vi "Stop Live Mode.vi"(7 "Close Viewer":bool=TRUE, 8 "error in (no error)":errorcluster, 10 "Mode":T1, 11 "Application in":refnum<class "Application.lvclass">) -> (0 "error out":errorcluster, 3 "Application out":refnum<class "Application.lvclass">)   [LabVIEW 2023, in "Application.lvlib" / "Application.lvclass"]
uses:
  Application.lvclass
  Application.lvclass/Application.ctl
  Hardware/Camera Messages/Stop Live Mode Msg/Stop Live Mode Msg.lvclass
  Hardware/Sync Device Messages/Stop Streaming Msg/Stop Streaming Msg.lvclass
  Mode.ctl
  Application.lvlib
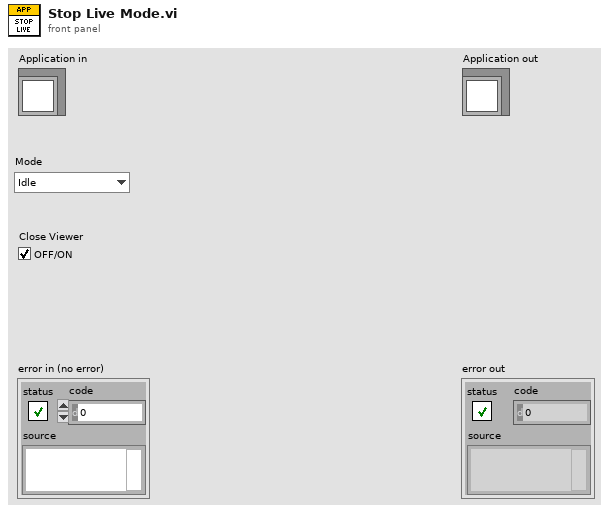
[diagram p1: front panel]
types:
  T1 = typedef "Application.lvlib/Mode.ctl" = enum16{"Idle", "Cancel", "Live", "Stream", "Autofocus", "Z-Stack"}
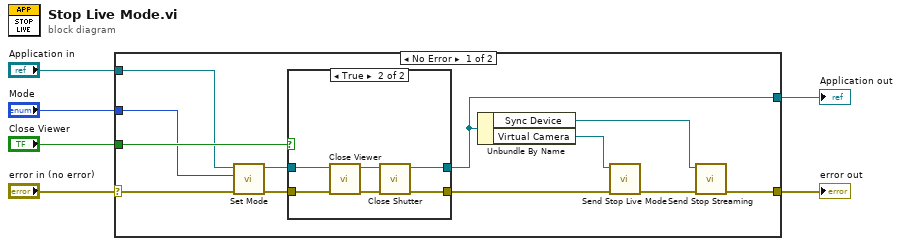
[diagram p0: block diagram]
diagram:
  n1 = case shown="No Error" "error in (no error)" {
    selector: "error in (no error)" -> [w13 w28]
    tunnel: [w9 w28] -> w5
    tunnel: [w17 w27] -> w3
    tunnel: "Application in" -> [w14 w27]
    tunnel: "Close Viewer" -> [w18 _]
    tunnel: "Mode" -> [w12 _]
    frame No Error {
      n2 = call-dynamic "Set Mode.vi"("error in (no error)"=w13, "New Mode"=w12, "Application in"=w14) -> ("error out"=w16:errorcluster, "Application out"=w15:refnum<class "Application.lvclass">)  [unwired: 7 in]
      n3 = case shown="True" w18 {
        tunnel: w16 -> [w19 w26]
        tunnel: w15 -> [w20 w25]
        tunnel: [w20 w22] -> w17
        tunnel: [w19 w21] -> w11
        frame False {
        }
        frame True {
          n4 = call-dynamic "Close Viewer.vi"("error in (no error)"=w26, "Application in"=w25) -> ("error out"=w23:errorcluster, "Application out"=w24:refnum<class "Application.lvclass">)  [unwired: 8 in]
          n5 = call-dynamic "Close Shutter.vi"("error in (no error)"=w23, "Application in"=w24) -> ("error out"=w21:errorcluster, "Application out"=w22:refnum<class "Application.lvclass">)  [unwired: 8 in]
        }
      }
      n6 = Unbundle By Name(w17) -> ("Sync Device"=w7:refnum<class "Message Enqueuer.lvclass">, "Virtual Camera"=w10:refnum<class "Message Enqueuer.lvclass">)
      n7 = call "Send Stop Live Mode.vi"("error in (no error)"=w11, "Message Enqueuer"=w10) -> ("error out"=w8:errorcluster)  [unwired: 8 in, 1 out]
      n8 = call "Send Stop Streaming.vi"("error in (no error)"=w8, "Message Enqueuer"=w7) -> ("error out"=w9:errorcluster)  [unwired: 8 in, 1 out]
    }
    frame Error {
    }
  }
  "error out" <- w5
  "Application out" <- w3
